vi "Joystick Control.vi"(8 "error in (no error)":errorcluster, 11 "controller in":refnum<k24>) -> (0 "error out":errorcluster, 3 "controller out":refnum<k24>)   [LabVIEW 2011]
uses:
  C:/Users/Admin/Desktop/Gantry Code Transfer/source/Code Transfer/Aerotech.A3200.dll
  Aerotech.A3200.dll
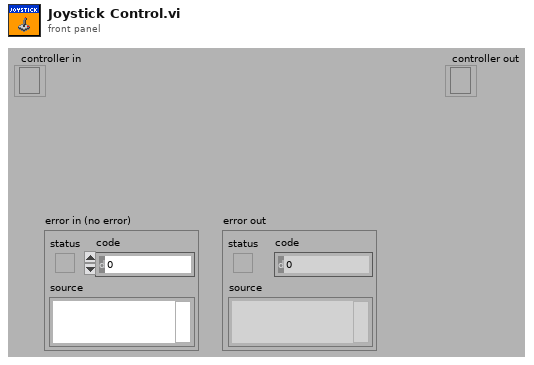
[diagram p1: front panel]
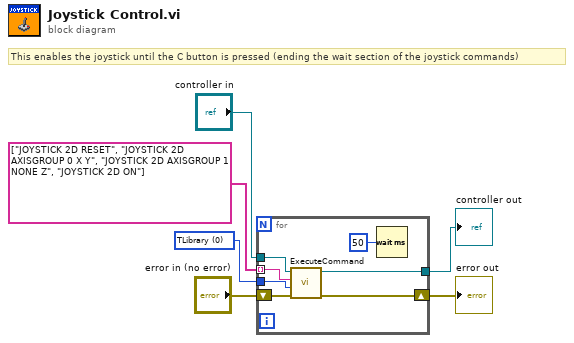
[diagram p0: block diagram]
diagram:
  w4 = 0 items=["TLibrary", "T01", "T02", "T03", "T04", "T05", "T06", "T07", "T08", "T09", "T10", "T11", "T12", "T13", "T14", "T15", "T16", "T17", "T18", "T19", "T20", "T21", "T22", "T23", "T24", "T25", "T26", "T27", "T28", "T29", "T30", "T31"] ("taskId")
  # "This enables the joystick until the C button is pressed (ending the wait section of the joystick commands)"
  n1 = for {
    shift-right: [w12] -> w5
    shift-left: "error in (no error)" -> [w13]
    tunnel: w4 -> [w9]
    tunnel: "controller in" -> [w11]
    tunnel: [w10] -> w2
    tunnel: string[] ["JOYSTICK 2D RESET", "JOYSTICK 2D AXISGROUP 0 X Y", "JOYSTICK 2D AXISGROUP 1 NONE Z", "JOYSTICK 2D ON"] -> [w8] mode=indexing
    n2 = call "ExecuteCommand.vi"("error in (no error)"=w13, "taskId"=w9, "Command Code"=w8, "controller in"=w11) -> ("error out"=w12:errorcluster, "controller out"=w10:refnum<k24>)  [unwired: 5 in, 1 out]
    n3 = Wait (ms)(milliseconds to wait=u32 50) -> ()  [unwired: 1 out]
  }
  "error out" <- w5
  "controller out" <- w2
